vi "SLSC Get EDS Module Information.vi"(5 "Password":string, 7 "Username":string="admin", 8 "error in (no error)":errorcluster, 10 "Slot #":u32=4, 11 "Chassis IP Address":string) -> (0 "error out":errorcluster, 1 "SLSC Module Name":string, 2 "Initialized?":bool, 3 "SLSC EDS module":T1)   [LabVIEW 2020, in "SLSC EDS System Explorer.lvlib"]
doc: "This vi reads device tree from online SLSC module. If there is no connection possible it reads from a capabilities NVMEM .bin file. Then it creates a cluster containing the whole module tree."
uses:
  JSON parsing/EDSjsonStructure.ctl
  JSON parsing/enum.ctl
  JSON parsing/property.ctl
  JSON parsing/command.ctl
  JSON parsing/scale.ctl
  JSON parsing/physicalChannel.ctl
  JSON parsing/register.ctl
  System Explorer/SLSC EDS System Explorer.lvlib
  SLSC CD API/SLSC CD Engine/SLSC CD Engine.lvlib
  SLSC EDS API.lvlib
panel:
  # "not working\nregisterMap->registers->initialValue"
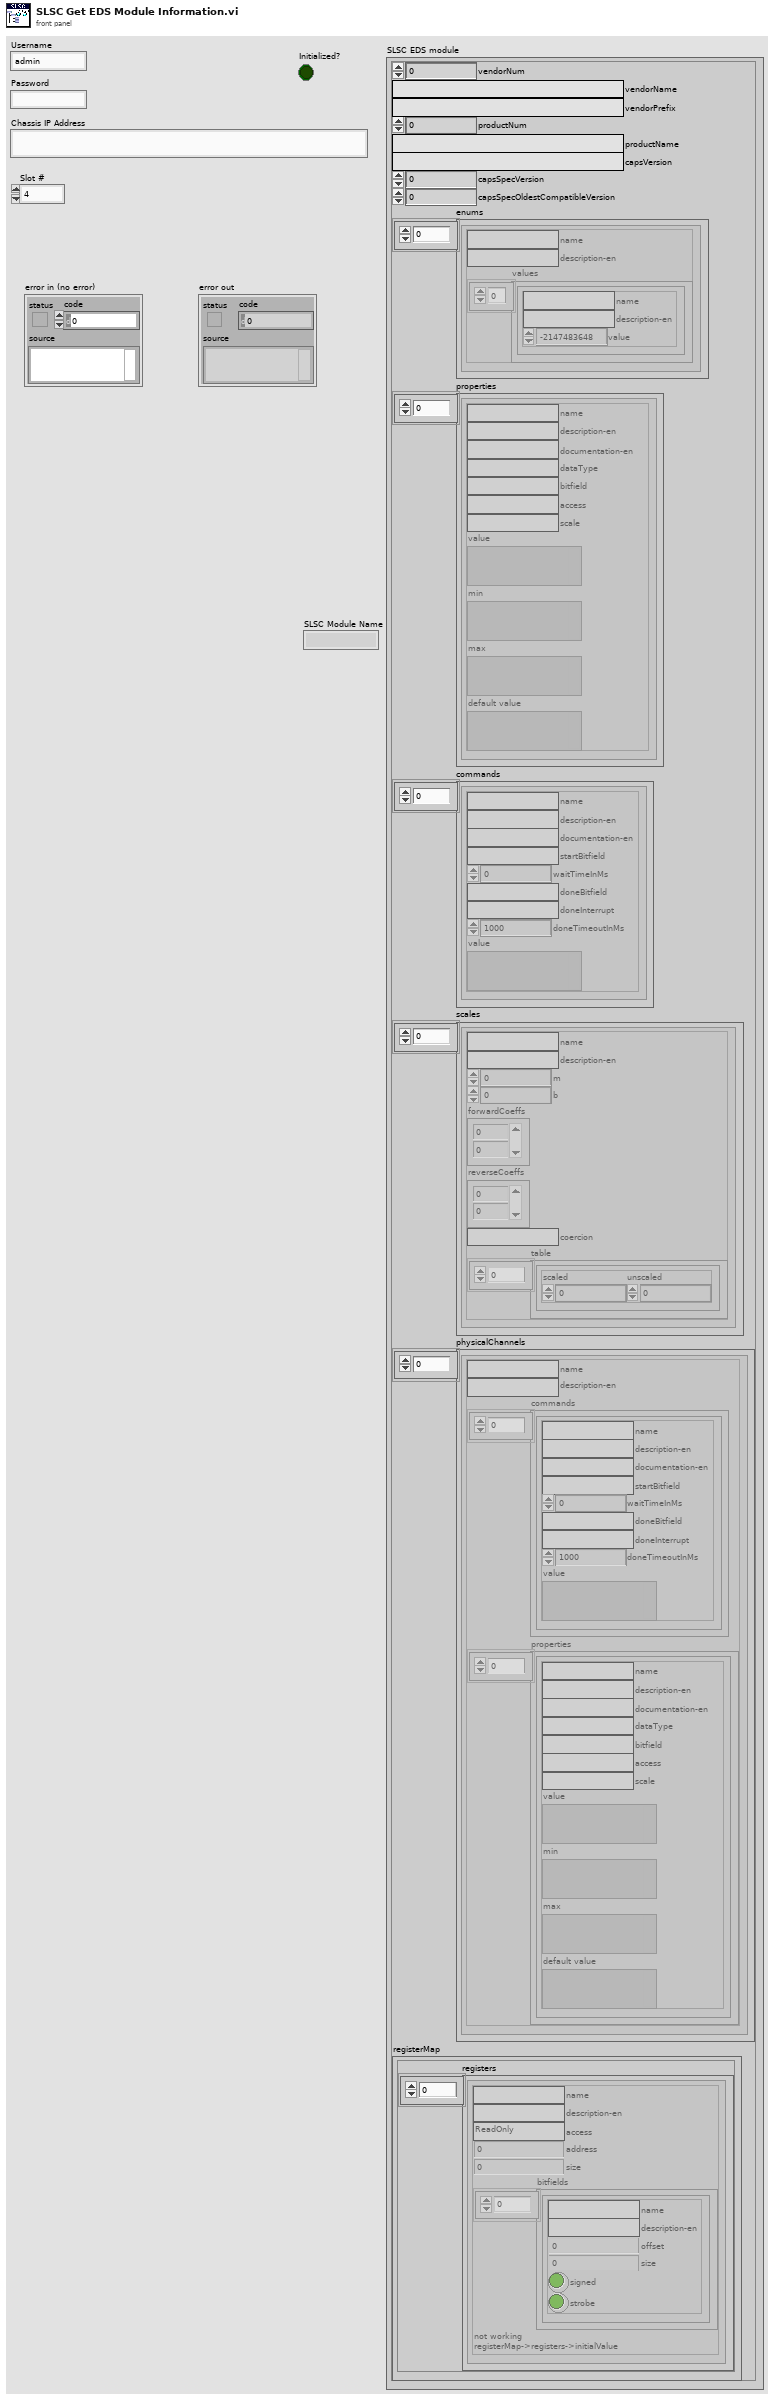
[diagram p1: front panel]
types:
  T1 = typedef "EDSjsonStructure.ctl" = cluster{"vendorNum":u32, "vendorName":string, "vendorPrefix":string, "productNum":u32, "productName":string, "capsVersion":string, "capsSpecVersion":u32, "capsSpecOldestCompatibleVersion":u32, "enums":T2[], "properties":T3[], "commands":T4[], "scales":T5[], "physicalChannels":T6[], "registerMap":cluster{"registers":T7[]}}
  T2 = typedef "enum.ctl" = cluster{"name":string, "description-en":string, "values":cluster{"name":string, "description-en":string, "value":i32}[]}
  T3 = typedef "property.ctl" = cluster{"name":string, "description-en":string, "documentation-en":string, "dataType":string, "bitfield":string, "access":string, "scale":string, "value":variant, "min":variant, "max":variant, "default value":variant}
  T4 = typedef "command.ctl" = cluster{"name":string, "description-en":string, "documentation-en":string, "startBitfield":string, "waitTimeInMs":i32, "doneBitfield":string, "doneInterrupt":string, "doneTimeoutInMs":i32, "value":variant}
  T5 = typedef "scale.ctl" = cluster{"name":string, "description-en":string, "m":dbl, "b":dbl, "forwardCoeffs":dbl[], "reverseCoeffs":dbl[], "coercion":string, "table":cluster{"scaled":dbl, "unscaled":dbl}[]}
  T6 = typedef "physicalChannel.ctl" = cluster{"name":string, "description-en":string, "commands":T4[], "properties":T3[]}
  T7 = typedef "register.ctl" = cluster{"name":string, "description-en":string, "access":string, "address":u32, "size":u32, "bitfields":cluster{"name":string, "description-en":string, "offset":u32, "size":u32, "signed":bool, "strobe":bool}[]}
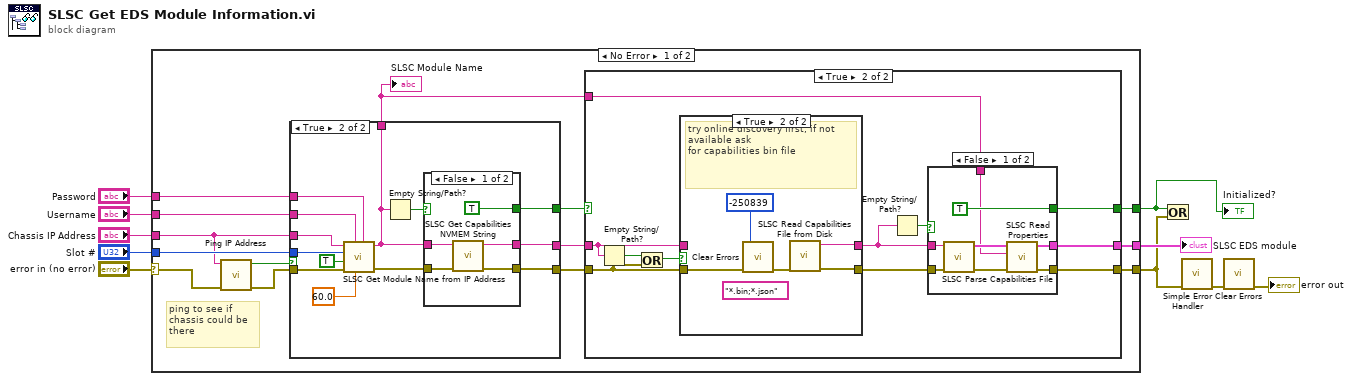
[diagram p0: block diagram]
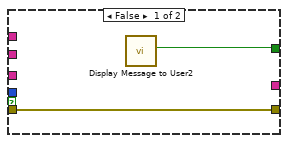
[diagram p5: hidden frame]
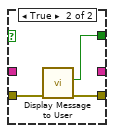
[diagram p6: hidden frame]
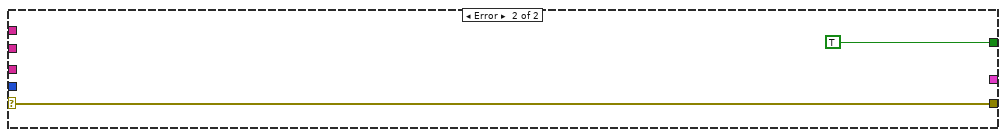
[diagram p7: hidden frame]
diagram:
  n1 = case shown="No Error" "error in (no error)" {
    selector: "error in (no error)" -> [w21 w77]
    tunnel: [w14 w77] -> w4
    tunnel: "Chassis IP Address" -> [w20 _]
    tunnel: "Slot #" -> [w24 _]
    tunnel: "Username" -> [w23 _]
    tunnel: "Password" -> [w22 _]
    tunnel: [w15 _] -> w5
    tunnel: [w11 TRUE ("Failed?")] -> w1
    frame No Error {
      # "ping to see if \nchassis could be \nthere"
      n2 = call "Ping IP Address.vi"("error in"=w21, "host"=w20) -> ("error out"=w19:errorcluster, "response?"=w18:bool)  [unwired: 7 in, 1 out]
      n3 = case shown="True" w18 {
        tunnel: w19 -> [w53 w58]
        tunnel: w20 -> [_ w64]
        tunnel: w24 -> [_ w63]
        tunnel: w23 -> [_ w66]
        tunnel: w22 -> [_ w65]
        tunnel: [w53 w62] -> w17
        tunnel: [_ w60] -> w16
        tunnel: [_ w57] -> w13
        tunnel: [w54 w59] -> w12
        frame False {
          n4 = call "Display Message to User2"() -> ("Yes"=w54:bool)  [unwired: 10 in, 1 out]
        }
        frame True {
          n5 = call "SLSC Get Module Name from IP Address.vi"("Password"=w65, "connect timeout"=60.0 ("connect timeout (10 sec)"), "Username"=w66, "Error In"=w58, "Wait for mDSN?"=TRUE, "Slot #"=w63, "Chassis IP Address"=w64) -> ("Error Out"=w56:errorcluster, "SLSC Module Name"=w57:string)  [unwired: 2 in, 1 out]
          n6 = Empty String/Path?(string/path=w57) -> (empty?=w61:bool)
          n7 = case shown="False" w61 {
            tunnel: w56 -> [w72 w75]
            tunnel: [w71 w74] -> w62
            tunnel: [w70 _] -> w60
            tunnel: w57 -> [w69 _]
            tunnel: [TRUE ("Yes") w73] -> w59
            frame False {
              n8 = call "SLSC Get Capabilities NVMEM String.vi"("error in (no error)"=w72, "SLSC Device"=w69) -> ("error out"=w71:errorcluster, "capabilities NVMEM"=w70:string)  [unwired: 8 in]
            }
            frame True {
              n9 = call "Display Message to User"("error in (no error)"=w75) -> ("error out"=w74:errorcluster, "Yes"=w73:bool)  [unwired: 9 in]
            }
          }
        }
      }
      "SLSC Module Name" <- w13
      n10 = case shown="True" w12 {
        tunnel: w17 -> [w25 w31]
        tunnel: w16 -> [_ w30]
        tunnel: [_ w35] -> w15
        tunnel: [w25 w34] -> w14
        tunnel: w13 -> [_ w33]
        tunnel: [_ w26] -> w11
        frame False {
        }
        frame True {
          n11 = Empty String/Path?(string/path=w30) -> (empty?=w29:bool)
          n12 = Or(x=w29, y=w31) -> (x .or. y?=w32:bool)
          n13 = case shown="True" w32 {
            tunnel: [w46 w50] -> w36
            tunnel: w30 -> [w47 _]
            tunnel: [w47 w49] -> w28
            tunnel: w31 -> [w46 w48]
            frame False {
            }
            frame True {
              (unwired) "*.bin;*.json" ("pattern (all files)")
              # "try online discovery first, if not available ask \nfor capabilities bin file"
              n14 = call <vilib>:"Clear Errors.vi"("error in (no error)"=w48, "specific error code to clear (0: all)"=-250839) -> ("error out"=w51:errorcluster)  [unwired: 4 in, 1 out]
              n15 = call "SLSC Read Capabilities File from Disk.vi"("error in (no error)"=w51) -> ("error out"=w50:errorcluster, "Capability file"=w49:string)  [unwired: 9 in]
            }
          }
          n16 = Empty String/Path?(string/path=w28) -> (empty?=w27:bool)
          n17 = case shown="False" w27 {
            tunnel: w36 -> [w44 w45]
            tunnel: [w41 _] -> w35
            tunnel: [w40 w45] -> w34
            tunnel: w33 -> [w37 _]
            tunnel: w28 -> [w39 _]
            tunnel: [TRUE _] -> w26
            frame False {
              n18 = call "SLSC Parse Capabilities File.vi"("error in"=w44, "module capabilities JSON string"=w39) -> ("error out"=w42:errorcluster, "SLSC EDS module"=w43:T1)  [unwired: 7 in, 1 out]
              n19 = call "SLSC Read Properties.vi"("error in (no error)"=w42, "SLSC Device"=w37, "SLSC EDS module in"=w43) -> ("error out"=w40:errorcluster, "SLSC EDS module out"=w41:T1)  [unwired: 7 in]
            }
            frame True {
            }
          }
        }
      }
    }
    frame Error {
    }
  }
  "SLSC EDS module" <- w5
  "Initialized?" <- w1
  n20 = Or(x=w1, y=w4) -> ()  [unwired: 1 out]
  n21 = call <vilib>:"Simple Error Handler.vi"("error in (no error)"=w4) -> ("error out"=w3:errorcluster)  [unwired: 4 in, 4 out]
  n22 = call <vilib>:"Clear Errors.vi"("error in (no error)"=w3) -> ("error out"=→"error out":errorcluster)  [unwired: 5 in, 1 out]
